vi "connection open schema.vi"(7 "Schema":i32(ring)=-1 items=["adSchemaProviderSpecific"=-1, "adSchemaAsserts"=0, "adSchemaCatalogs"=1, "adSchemaCharacterSets"=2, "adSchemaCollations"=3, "adSchemaColumns"=4, "adSchemaCheckConstraints"=5, "adSchemaConstraintColumnUsage"=6, "adSchemaConstraintTableUsage"=7, "adSchemaKeyColumnUsage"=8, "adSchemaReferentialContraints, adSchemaReferentialConstraints"=9, "adSchemaTableConstraints"=10, "adSchemaColumnsDomainUsage"=11, "adSchemaIndexes"=12, "adSchemaColumnPrivileges"=13, "adSchemaTablePrivileges"=14, "adSchemaUsagePrivileges"=15, "adSchemaProcedures"=16, "adSchemaSchemata"=17, "adSchemaSQLLanguages"=18, "adSchemaStatistics"=19, "adSchemaTables"=20, "adSchemaTranslations"=21, "adSchemaProviderTypes"=22, "adSchemaViews"=23, "adSchemaViewColumnUsage"=24, "adSchemaViewTableUsage"=25, "adSchemaProcedureParameters"=26, "adSchemaForeignKeys"=27, "adSchemaPrimaryKeys"=28, "adSchemaProcedureColumns"=29, "adSchemaDBInfoKeywords"=30, "adSchemaDBInfoLiterals"=31, "adSchemaCubes"=32, "adSchemaDimensions"=33, "adSchemaHierarchies"=34, "adSchemaLevels"=35, "adSchemaMeasures"=36, "adSchemaProperties"=37, "adSchemaMembers"=38, "adSchemaTrustees"=39], 8 "error in (no error)":errorcluster, 9 "Fields":string[](array[string]), 10 "Restrictions":string[][](array[string]), 11 "ADODB._Connection":refnum<k7>) -> (0 "error out":errorcluster, 1 "Schema Out":string[][](array[string]), 2 "Fields Out":string[](array[string]), 3 "ADODB._Connection":refnum<k7>)   [LabVIEW 2020]
uses:
  <userlib>/_OpenG.lib/array/array.llb/Filter 1D Array (String)__ogtk.vi
  <userlib>/_OpenG.lib/array/array.llb/Index 1D Array Elements (String)__ogtk.vi
  <userlib>/_OpenG.lib/array/array.llb/Filter 1D Array with Scalar (String)__ogtk.vi
  <vilib>/addons/database/_DB Variant To Data/Database Variant To Data.xnode
panel:
  # "-Each column contains rows: (fieldname; value).\n-Multiple fieldnames (columns) can be passed\n-The same fieldname can be passed with different values (as different columns)\n-If any value in the recordset matches for a given field, the restriction is met\n-If any field does not meet a restriction, the recordset row is not passed\n-Otherwise, the recordset row is always passed\nNOTE: Unlike ADO.NET OpenSchema restrictions arguement, the restrictions 2d array is an array of field names and values. If I figure out how to use the OpenSchema method Restrictions directly,\nthe Restrictions will be changed to match the ADO.NET dolumentation"
  # "Return a table with the specified field names. If empty, return all fields."
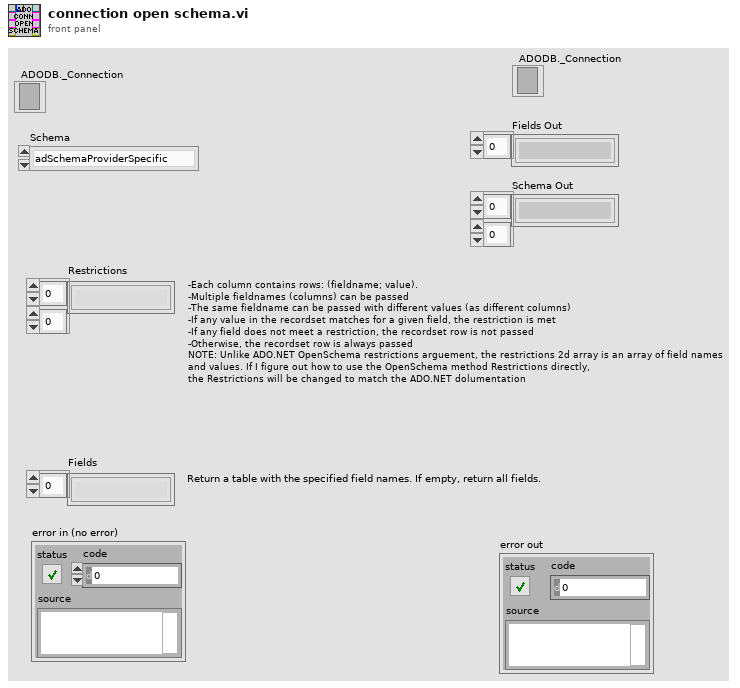
[diagram p1: front panel]
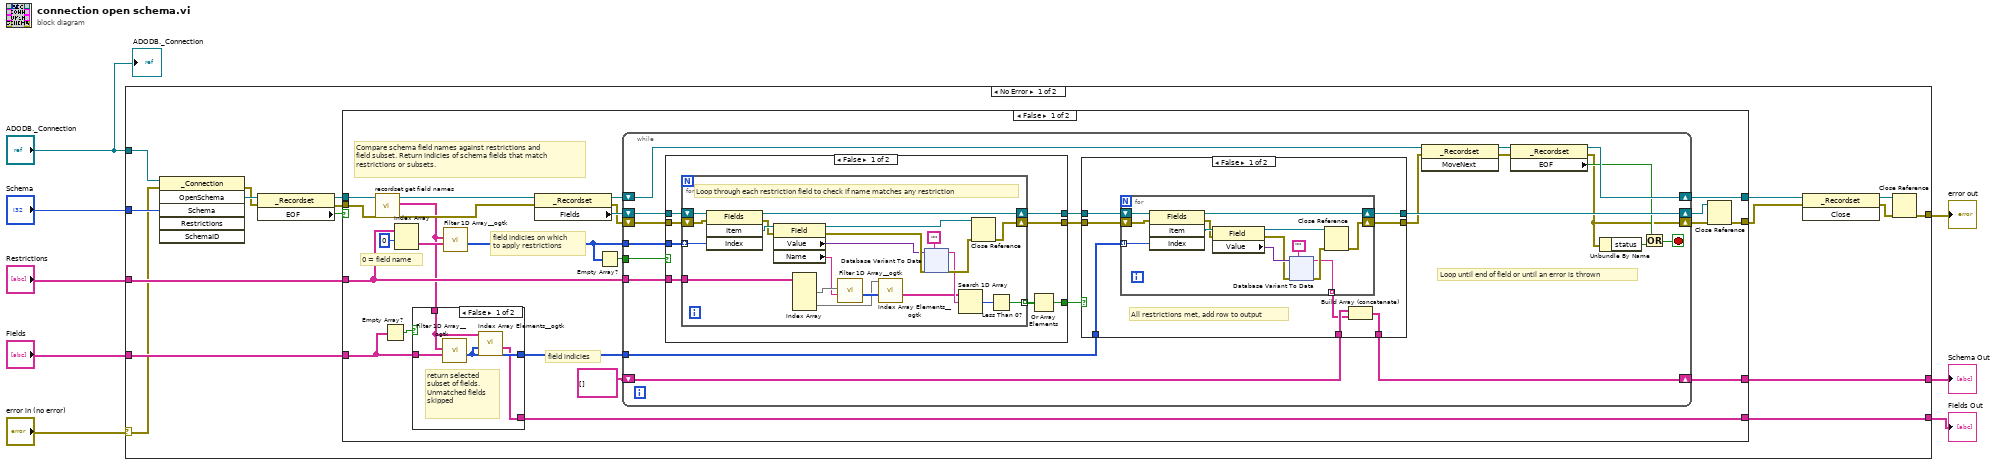
[diagram p0: block diagram]
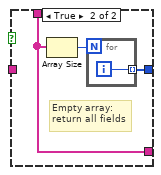
[diagram p2: hidden frame]
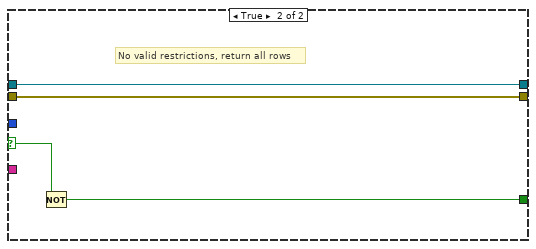
[diagram p3: hidden frame]
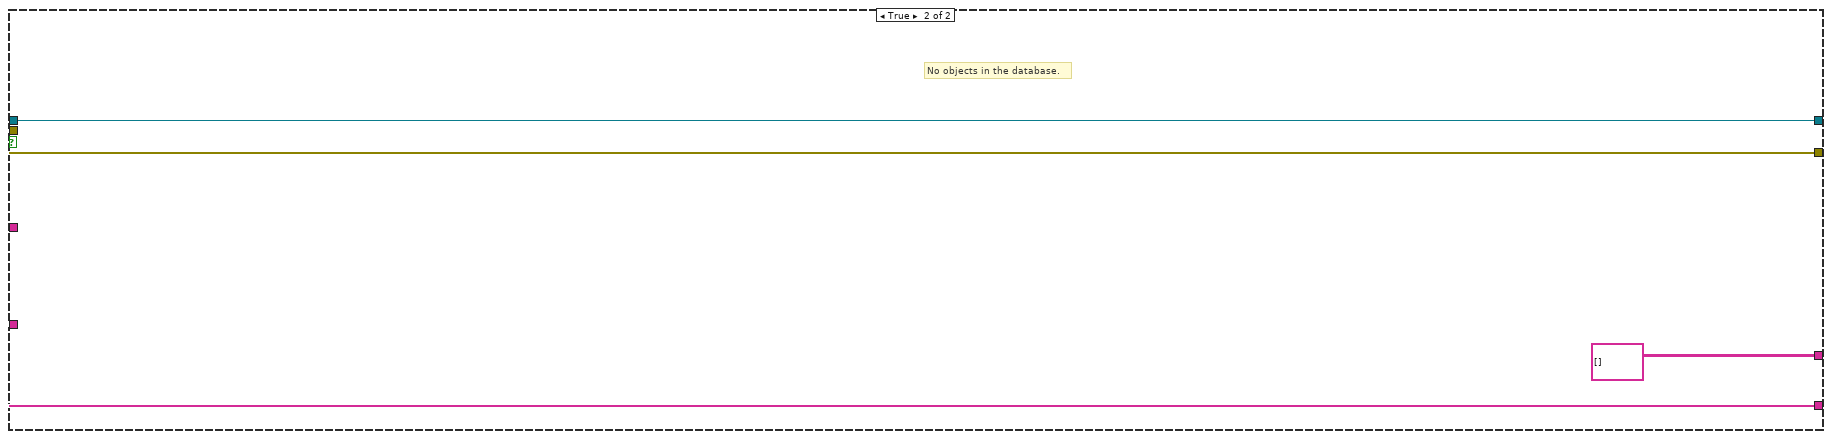
[diagram p5: hidden frame]
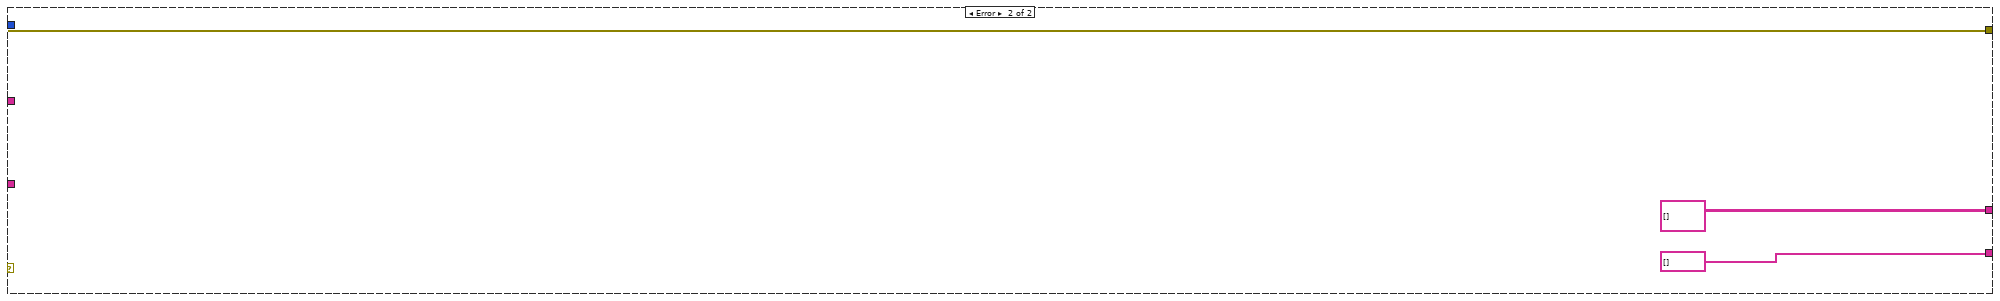
[diagram p6: hidden frame]
diagram:
  n1 = case shown="No Error" "error in (no error)" {
    selector: "error in (no error)" -> [w13 w205]
    tunnel: "ADODB._Connection" -> [w25 _]
    tunnel: "Schema" -> [w24 _]
    tunnel: "Restrictions" -> [w20 _]
    tunnel: "Fields" -> [w19 _]
    tunnel: [w16 string[] [] ("Fields")] -> w5
    tunnel: [w15 string[][] []] -> w4
    tunnel: [w14 w205] -> w3
    frame No Error {
      n2 = invoke class="_Connection" method="OpenSchema"(reference=w25, error in=w13, "Schema"=w24) -> (error out=w17:errorcluster, "OpenSchema"=w23:refnum<k7>)  [unwired: 3 in, 4 out]
      n3 = property class="_Recordset"(reference=w23, error in=w17) -> (reference out=w21:refnum<k7>, error out=w18:errorcluster, "EOF"=w22:bool)
      n4 = case shown="False" w22 {
        tunnel: [w45 string[][] []] -> w15
        tunnel: [w42 w200] -> w12
        tunnel: [w40 w202] -> w11
        tunnel: w21 -> [w39 w202]
        tunnel: w20 -> [w35 _]
        tunnel: w19 -> [w28 w199]
        tunnel: w18 -> [w33 w200]
        tunnel: [w26 w199] -> w16
        frame False {
          # "field indicies"
          # "Compare schema field names against restrictions and\nfield subset. Return indicies of schema fields that match\nrestrictions or subsets."
          # "field indicies on which\nto apply restrictions"
          # "0 = field name"
          n5 = call "recordset get field names.vi"("error in (no error)"=w33, "recordset in"=w39) -> ("error out"=w34:errorcluster, "field names"=w30:string[], "recordset out"=w36:refnum<k7>)  [unwired: 7 in]
          n6 = Empty Array?(array=w28) -> (empty?=w27:bool)
          n7 = Index Array(array=w35, index (row)=0) -> (element=w37:string[])  [unwired: 1 in]
          n8 = case shown="False" w27 {
            tunnel: w30 -> [w52 w53]
            tunnel: [w51 w55] -> w29
            tunnel: w28 -> [w50 _]
            tunnel: [w49 w53] -> w26
            frame False {
              # "return selected subset of fields.\nUnmatched fields skipped"
              n9 = call-poly <userlib>:"Filter 1D Array__ogtk.vi"("items to filter"=w50, "array"=w52) -> ("filtered item indices"=w51:i32[])  [unwired: 4 in, 1 out]
              n10 = call-poly <userlib>:"Index Array Elements__ogtk.vi"("indices"=w51, "array"=w52) -> ("elements"=w49:string[])  [unwired: 9 in]
            }
            frame True {
              # "Empty array:\nreturn all fields"
              n11 = Array Size(array=w53) -> (size(s)=w54:i32)
              n12 = for {
                N: w54 -> [_]
                tunnel: [w56] -> w55 mode=indexing
                i -> [w56]
              }
            }
          }
          n13 = call-poly <userlib>:"Filter 1D Array__ogtk.vi"("items to filter"=w37, "array"=w30) -> ("filtered item indices"=w31:i32[])  [unwired: 4 in, 1 out]
          n14 = property class="_Recordset"(reference=w36, error in=w34) -> (reference out=w48:refnum<k7>, error out=w46:errorcluster, "Fields"=w47:refnum<k7>)
          n15 = Empty Array?(array=w31) -> (empty?=w32:bool)
          n16 = while {
            shift-right: [w69] -> w41
            shift-left: w47 -> [w77]
            shift-right: [w67] -> w43
            shift-left: w46 -> [w75]
            shift-right: [w72] -> w40
            shift-left: w48 -> [w65]
            shift-right: [w58] -> w45
            shift-left: string[][] [] -> [w59]
            tunnel: w31 -> [w64]
            tunnel: w35 -> [w63]
            tunnel: w29 -> [w61]
            tunnel: w32 -> [w57]
            stop <- w76 stop-if-true
            # "Loop until end of field or until an error is thrown"
            n17 = case shown="False" w57 {
              selector: w57 -> [_ w142]
              tunnel: w77 -> [w85 w140]
              tunnel: w75 -> [w84 w139]
              tunnel: [w83 w140] -> w70
              tunnel: w64 -> [w82 _]
              tunnel: w63 -> [w81 _]
              tunnel: [w79 w141] -> w62
              tunnel: [w78 w139] -> w60
              frame False {
                n18 = for {
                  shift-right: [w104] -> w83
                  shift-left: w85 -> [w106]
                  shift-right: [w97] -> w78
                  shift-left: w84 -> [w105]
                  tunnel: w82 -> [w95] mode=indexing
                  tunnel: w81 -> [w94]
                  tunnel: [w90] -> w80 mode=indexing
                  # "Loop through each restriction field to check if name matches any restriction"
                  n19 = invoke class="Fields" method="Item"(reference=w106, error in=w105, "Index"=w95) -> (reference out=w104:refnum<k7>, error out=w96:errorcluster, "Item"=w103:refnum<k7>)  [unwired: 1 in, 1 out]
                  n20 = property class="Field"(reference=w103, error in=w96) -> (reference out=w99:refnum<k7>, error out=w101:errorcluster, "Value"=w100:variant, "Name"=w86:string)
                  n21 = Index Array(array=w94) -> (element #1=w93:string[], element #2=w88:string[])  [unwired: 4 in]
                  n22 = call-poly <userlib>:"Filter 1D Array__ogtk.vi"("items to filter"=w86, "array"=w93) -> ("filtered item indices"=w89:i32[])  [unwired: 4 in, 1 out]
                  n23 = call-poly <userlib>:"Index Array Elements__ogtk.vi"("indices"=w89, "array"=w88) -> ("elements"=w87:string[])  [unwired: 9 in]
                  n24 = xnode "Database Variant To Data"("database variant"=w100, "error in"=w101, "type"="") -> ("data"=w92:string, "error out"=w98:errorcluster)
                  n25 = Search 1D Array(1D array=w87, element=w92) -> (index of element=w91:i32)  [unwired: 1 in]
                  n26 = Close Reference(reference=w99, error in (no error)=w98) -> (error out=w97:errorcluster)
                  n27 = Less Than 0?(x=w91) -> (x < 0?=w90:bool)
                }
                n28 = Or Array Elements(Boolean array=w80) -> (logical OR=w79:bool)
              }
              frame True {
                # "No valid restrictions, return all rows"
                n29 = Not(x=w142) -> (.not. x?=w141:bool)
              }
            }
            n30 = case shown="False" w62 {
              tunnel: w70 -> [w150 w197]
              tunnel: [w149 w197] -> w69
              tunnel: [w148 w196] -> w66
              tunnel: w61 -> [w146 _]
              tunnel: w60 -> [w147 w196]
              tunnel: w59 -> [w145 w198]
              tunnel: [w143 w198] -> w58
              frame False {
                # "All restrictions met, add row to output"
                n31 = for {
                  shift-right: [w162] -> w149
                  shift-left: w150 -> [w163]
                  shift-right: [w161] -> w148
                  shift-left: w147 -> [w160]
                  tunnel: w146 -> [w152] mode=indexing
                  tunnel: [w151] -> w144 mode=indexing
                  n32 = invoke class="Fields" method="Item"(reference=w163, error in=w160, "Index"=w152) -> (reference out=w162:refnum<k7>, error out=w157:errorcluster, "Item"=w158:refnum<k7>)  [unwired: 1 in, 1 out]
                  n33 = property class="Field"(reference=w158, error in=w157) -> (reference out=w153:refnum<k7>, error out=w155:errorcluster, "Value"=w156:variant)
                  n34 = xnode "Database Variant To Data"("database variant"=w156, "error in"=w155, "type"="") -> ("data"=w151:string, "error out"=w154:errorcluster)
                  n35 = Close Reference(reference=w153, error in (no error)=w154) -> (error out=w161:errorcluster)
                }
                n36 = Build Array (concatenate)(w145, w144) -> (w143:string[][])
              }
              frame True {
                # "At least one restriction was not met, skip adding row"
              }
            }
            n37 = invoke class="_Recordset" method="MoveNext"(reference=w65, error in=w66) -> (reference out=w74:refnum<k7>, error out=w73:errorcluster)  [unwired: 1 in, 1 out]
            n38 = property class="_Recordset"(reference=w74, error in=w73) -> (reference out=w72:refnum<k7>, error out=w67:errorcluster, "EOF"=w68:bool)
            n39 = Unbundle By Name(w67) -> ("status"=w71:bool)
            n40 = Or(x=w68, y=w71) -> (x .or. y?=w76:bool)
          }
          n41 = Close Reference(reference=w41, error in (no error)=w43) -> (error out=w42:errorcluster)
        }
        frame True {
          # "No objects in the database."
        }
      }
      n42 = invoke class="_Recordset" method="Close"(reference=w11, error in=w12) -> (reference out=w10:refnum<k7>, error out=w9:errorcluster)  [unwired: 1 in, 1 out]
      n43 = Close Reference(reference=w10, error in (no error)=w9) -> (error out=w14:errorcluster)
    }
    frame Error {
    }
  }
  "Fields Out" <- w5
  "Schema Out" <- w4
  "error out" <- w3
  "ADODB._Connection" <- "ADODB._Connection"
